vi "trim.vi"(1 "Down":bool, 2 "Up":bool) -> (0 "Trim":dbl)   [LabVIEW 2014]
uses:
  Robot Global Data.vi
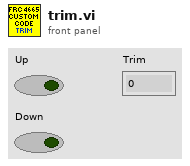
[diagram p1: front panel]
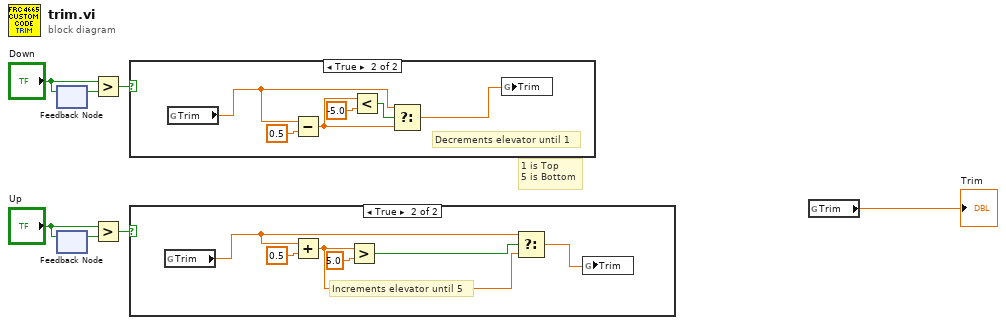
[diagram p0: block diagram]
diagram:
  # "1 is Top\n5 is Bottom"
  n1 = feedback #1() -> (w5:bool)  [unwired: 1 in]
  n2 = feedback-in #1("Down") -> ()
  n3 = feedback #2() -> (w7:bool)  [unwired: 1 in]
  n4 = feedback-in #2("Up") -> ()
  n5 = Greater?(x="Down", y=w5) -> (0:w4:bool)
  n6 = Greater?(x="Up", y=w7) -> (0:w6:bool)
  n7 = case shown="True" w4 {
    frame False {
    }
    frame True {
      # "Decrements elevator until 1"
      n8 = global read "Robot Global Data.vi" "Trim"() -> (w9:dbl)
      n9 = Subtract(x=w9, y=0.5) -> (x-y=w11:dbl)
      n10 = Less?(x=w11, y=-5.0) -> (x < y?=w12:bool)
      n11 = Select(t=w9, s=w12, f=w11) -> (s? t:f=w8:dbl)
      n12 = global write "Robot Global Data.vi" "Trim"(w8) -> ()
    }
  }
  n13 = case shown="True" w6 {
    frame False {
    }
    frame True {
      # "Increments elevator until 5"
      n14 = global read "Robot Global Data.vi" "Trim"() -> (w15:dbl)
      n15 = Add(x=w15, y=0.5) -> (x+y=w16:dbl)
      n16 = Greater?(x=w16, y=5.0) -> (0:w17:bool)
      n17 = Select(t=w15, s=w17, f=w16) -> (s? t:f=w14:dbl)
      n18 = global write "Robot Global Data.vi" "Trim"(w14) -> ()
    }
  }
  n19 = global read "Robot Global Data.vi" "Trim"() -> (→"Trim":dbl)
